vi "GUI_LeCroy64Xi.vi"() -> ()   [LabVIEW 2020]
uses:
  Shared/GUI_Template/GUI_master/tcp_new_data_event.ctl
  Shared/GUI_Template/GUI_master/tcp new data cluster.ctl
  <vilib>/Utility/miscctls.llb/LVCursorListTypeDef.ctl
  <vilib>/Utility/config.llb/Read Key (String).vi
  <vilib>/Waveform/WDTOps.llb/WDT Waveform Duration DBL.vi
  <vilib>/Analysis/NI_AAL_SigProc.lvlib
  <vilib>/measure/NI_MAPro.lvlib
  <vilib>/measure/mascope.llb/Amplitude and Levels 1 chan.vi
  <vilib>/measure/mascope.llb/Pulse Measurements 1 chan.vi
  <vilib>/Utility/config.llb/NI_LVConfig.lvlib
panel:
  in  "graph":bool
  in  "GUInumPoints::1":dbl=50000.0 caption="GUI num Points" min=100.0 max=10000.0 format="%#_6p"
  in  "TimeAxis.Time offset::1":dbl=0.0002 caption="Time offset (s)" min=-0.1 max=0.1 format="%#_6p"
  in  "Scale as scope":bool
  in  "Channel to scale":i32(ring)=1 items=["Channel 1", "Channel 2", "Channel 3", "Channel 4"]
  out "800nm w.r.t. Discharge (mean)":dbl format="%.1p"
  out "800nm w.r.t. 532nm":dbl format="%.1p"
  in  "Trigger.mode::1":u16(ring)=2 caption="Trigger mode" items=["Auto", "Normal", "Single", "Single, auto trigger"]
  in  "Trigger.Slope::1":u16(ring) caption="Trigger Slope" items=["Rising", "Falling"]
  in  "Trigger.Source::1":u16(ring)=1 caption="Trigger Source" items=["Channel 1", "Channel 2", "Channel 3", "Channel 4", "External", "Power Line"]
  in  "Trigger.Level::1":dbl=0.04 caption="Trigger Level (V)" min=0.0001 max=30.0 format="%#_6p"
  in  "TimeAxis.Max Sample Points::1":i32(ring)=5000 caption="Max Sample Points" items=["50"=50, "100"=100, "250"=250, "500"=500, "1000"=1000, "2500"=2500, "5K"=5000, "10K"=10000, "25K"=25000, "50K"=50000, "100K"=100000, "250K"=250000, "500K"=500000, "1M"=1000000, "2M"=2000000, "2.5M"=2500000, "5M"=5000000, "10M"=10000000, "25M"=25000000, "50M"=50000000, "100M"=100000000]
  in  "TimeAxis.Time base::1":dbl=0.0002 caption="Time base (s/div)" min=2e-10 max=1000.0 format="%#_6p"
  in  "Chenabled.Channel2::1":bool=TRUE caption="On/Off"
  in  "Verticaloffset.Channel2::1":dbl caption="Vertical Offset (V)" min=-40.0 max=40.0 format="%#.6p"
  in  "Bandwidth.Channel2::1":u16(ring) caption="Bandwidth" items=["Full", "20MHZ", "200MHZ"]
  in  "Verticalrange.Channel2::1":dbl=0.2 caption="Vertical Range (V)" min=0.0001 max=80.0 format="%#.6p"
  in  "Chenabled.Channel3::1":bool caption="On/Off"
  in  "Verticaloffset.Channel3::1":dbl caption="Vertical Offset (V)" min=-40.0 max=40.0 format="%#.6p"
  in  "Bandwidth.Channel3::1":u16(ring) caption="Bandwidth" items=["Full", "20MHZ", "200MHZ"]
  in  "Verticalrange.Channel3::1":dbl=0.2 caption="Vertical Range (V)" min=0.0001 max=80.0 format="%#.6p"
  in  "timeout::1":dbl caption="Timeout (ms)" min=0.0 max=10.0
  in  "Tab Control":T1(tab)
  out "all traces":waveform(dbl)[](graph)
  in  "value6::2":dbl=1.07e-07 caption="Dischage output" min=-9999999.0 max=9999999.0 step=1e-09 format="%#_6p"
  in  "value5::2":dbl=6e-08 caption="Dischage input" min=-9999999.0 max=9999999.0 step=1e-09 format="%#_6p"
  in  "value4::2":dbl=3e-09 caption="800nm diode" min=-9999999.0 max=9999999.0 step=1e-09 format="%#_6p"
  in  "value3::2":dbl caption="532nm diode" min=-9999999.0 max=9999999.0 step=1e-09 format="%#_6p"
  in  "Digitizer Traces":T2 caption="Raw Scope Data"
  in  "Type":enum16{"Peak fit", "Threshold"}[](array[ring])=[enum."Peak fit", enum."Threshold", enum."Peak fit", enum."Peak fit"]
  in  "Fit width":i32[](array[numeric])=[13, 15, 2000, 2000] min=3
  in  "Fit threshold":dbl[](array[numeric])=[0.02, 0.01, 0.02, 0.02]
  in  "Enable fitting":bool=TRUE
  in  "Enable fit cursors":bool=TRUE
  out "Number of peaks found":i32[](array[numeric])
  out "Time of peak":dbl[](array[numeric]) format="%.2p"
  in  "CH 4:":bool=TRUE
  in  "CH 3:":bool=TRUE
  in  "CH 2:":bool
  in  "CH 1:":bool
  in  "GUIdevice 1":string="LeCroy8254M"
  in  "GUIdevice 2":string="Offsets-Timing"
  out "error IO 2":errorcluster
  out "error":errorcluster
  out "tcp data event":T3
  out "duration":dbl format="%.2p"
  in  "Fit parameters file path":string="user data\\LeCroy_Fit_Parameters.txt"
  in  "stop":bool
  in  "Chenabled.Channel1::1":bool=TRUE caption="On/Off"
  in  "Verticaloffset.Channel1::1":dbl caption="Vertical Offset (V)" min=-5.0 max=5.0 format="%#.6p"
  in  "Bandwidth.Channel1::1":u16(ring) caption="Bandwidth" items=["Full", "20MHZ", "200MHZ"]
  in  "Verticalrange.Channel1::1":dbl=1.2 caption="Vertical Range (V)" min=0.0001 max=80.0 format="%#.6p"
  in  "Chenabled.Channel0::1":bool caption="On/Off"
  in  "Verticaloffset.Channel0::1":dbl caption="Vertical Offset (V)" min=-5.0 max=5.0 format="%#.6p"
  in  "Bandwidth.Channel0::1":u16(ring) caption="Bandwidth" items=["Full", "20MHZ", "200MHZ"]
  in  "Verticalrange.Channel0::1":dbl=0.2 caption="Vertical Range (V)" min=0.0001 max=80.0 format="%#.6p"
  # "Scope controls"
  # "Time axis"
  # "Scaling"
  # "Raw"
  # "Converted"
  # "Trigger"
  # "Channel 3"
  # "Channel 4"
  # "time offsets"
  # "time offsets"
  # "Fit settings"
  # "CH 1"
  # "CH 2"
  # "CH 3"
  # "CH 4"
  # "Fit output"
  # "CH 1"
  # "CH 2"
  # "CH 3"
  # "CH 4"
  # "Channel 2"
  # "Channel 1"
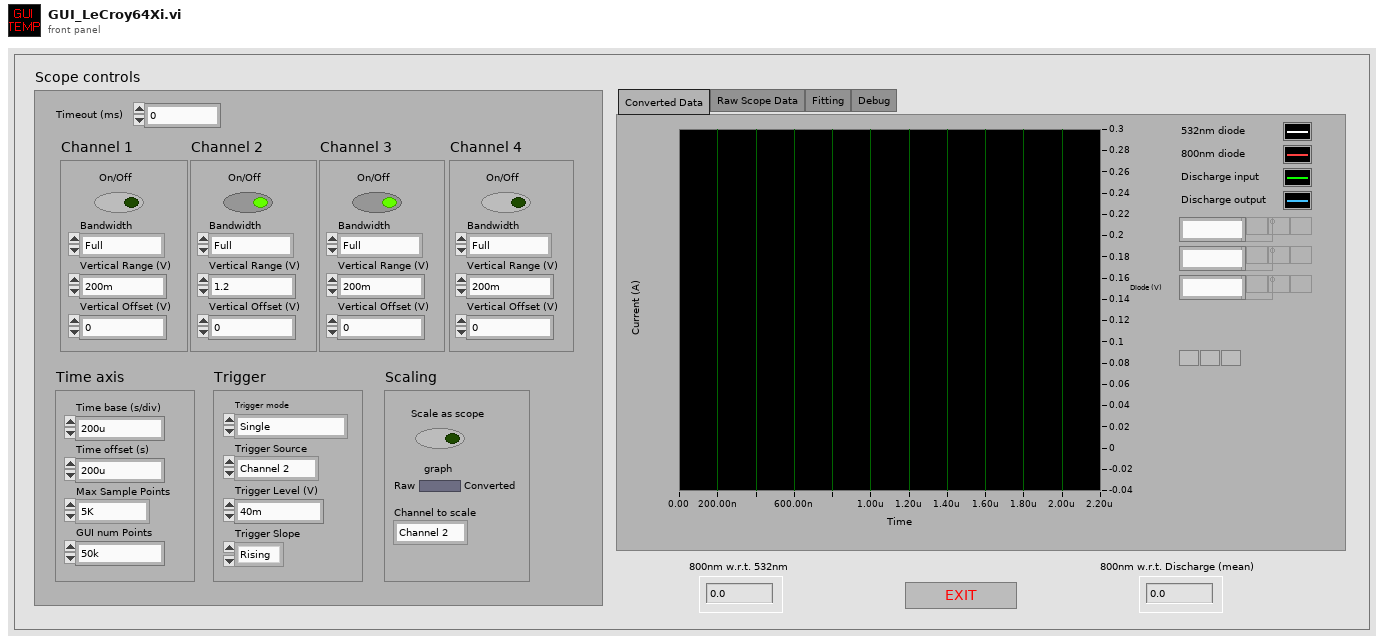
[diagram p1: front panel]
types:
  T1 = enum32{"Converted Data", "Raw Scope Data", "Fitting", "Debug"}
  T2 = cluster{"Channel::1":enum16{"Channel0", "Channel1", "Channel2", "Channel3"}, "scopeTraceGUI::1":waveform(dbl)[]}
  T3 = typedef "tcp_new_data_event.ctl" = refnum<user-event>
  T4 = typedef "tcp new data cluster.ctl" = cluster{"EventEnum":enum16{"new data", "connection status update"}, "Device name":string}
  T5 = enum32{"invalid app kind", "Development System", "Run Time System", "Student Edition", "Embedded LabVIEW", "Evaluation", "Custom"}
  T6 = enum32{"Invalid", "Standard", "Closed", "Hidden", "Minimized", "Maximized"}
  T7 = typedef "LVCursorListTypeDef.ctl" = cluster{"Name":string, "Color":u32, "Style":u8, "Point Style":u8, "Name Visible":bool, "Allow Drag":bool, "Cursor Mode":u32, "Plot":i32, "Index":i32, "Position":cluster{"X":dbl, "Y":dbl}, "X Scale":u32, "Y Scale":u32, "Watch Plots":i32[], "Watch All Plots":bool, "Plot Area":i32, "Label Offset":cluster{"X":dbl, "Y":dbl}}[]
  T8 = cluster{"Core":cluster{"Current VI Reference":refnum<vi>, "Close Panel on Exit?":bool}, "scopeTraceGUI::1":waveform(dbl)[], "Display Error Popup":bool, "time offsets":dbl[], "initilize fit":bool, "Fit peaks":dbl[], "fit cursors enabled":bool, "fitting enabled":bool}
  T9 = cluster{"Current VI Reference":refnum<vi>, "Close Panel on Exit?":bool}
  T10 = typedef "NI_LVConfig.lvlib/Config Data RefNum.ctl" = refnum<k1>
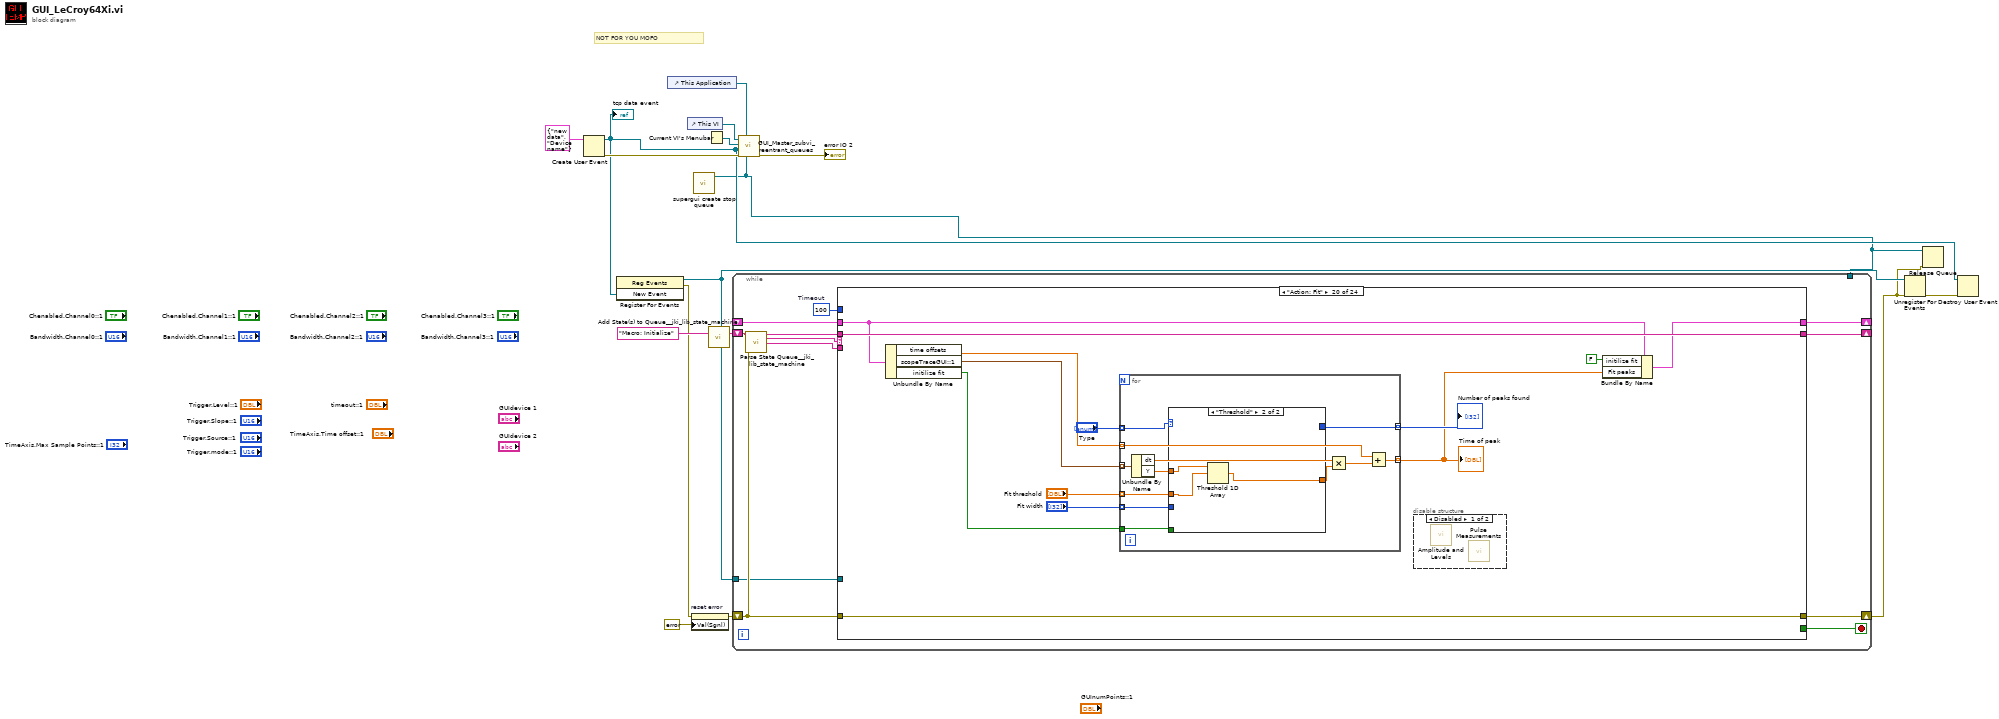
[diagram p0: block diagram]
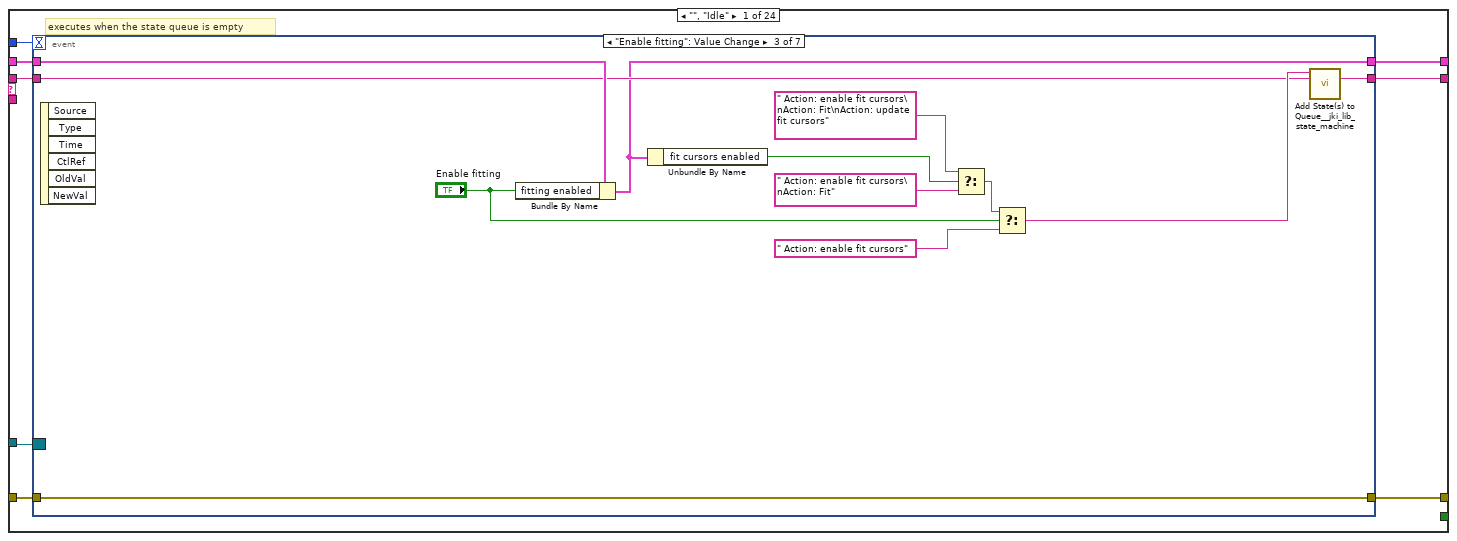
[diagram p2: hidden frame]
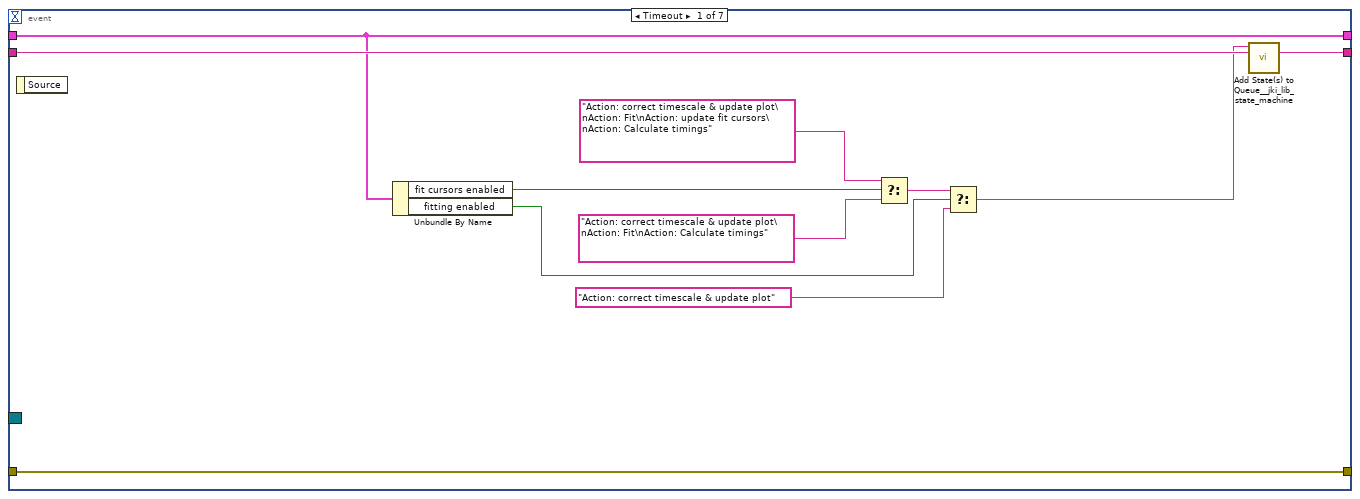
[diagram p3: hidden frame]
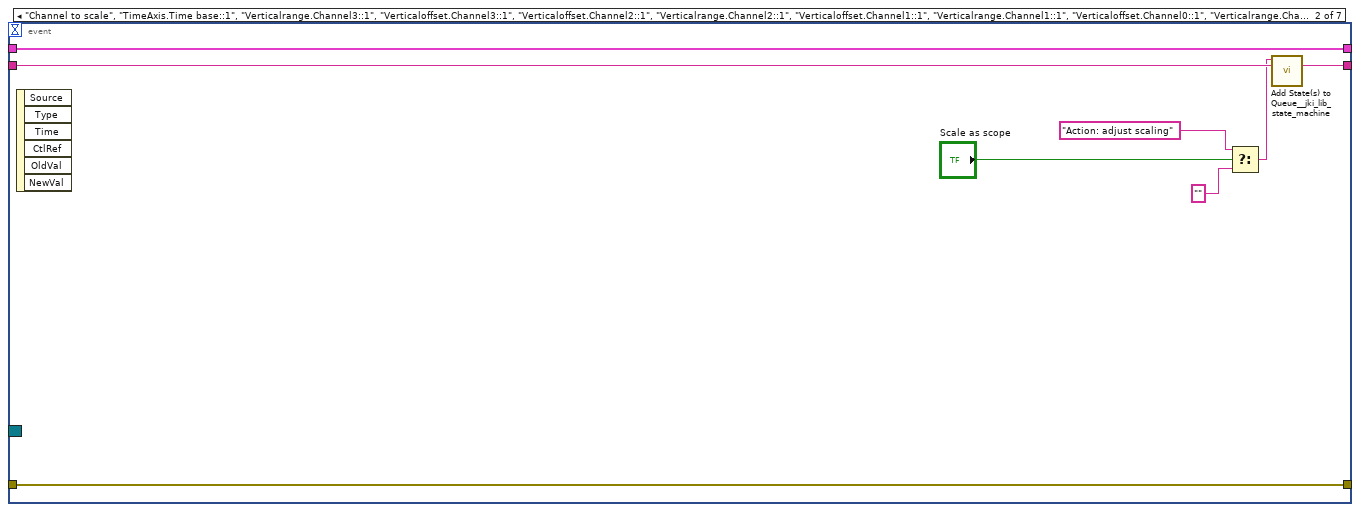
[diagram p4: hidden frame]
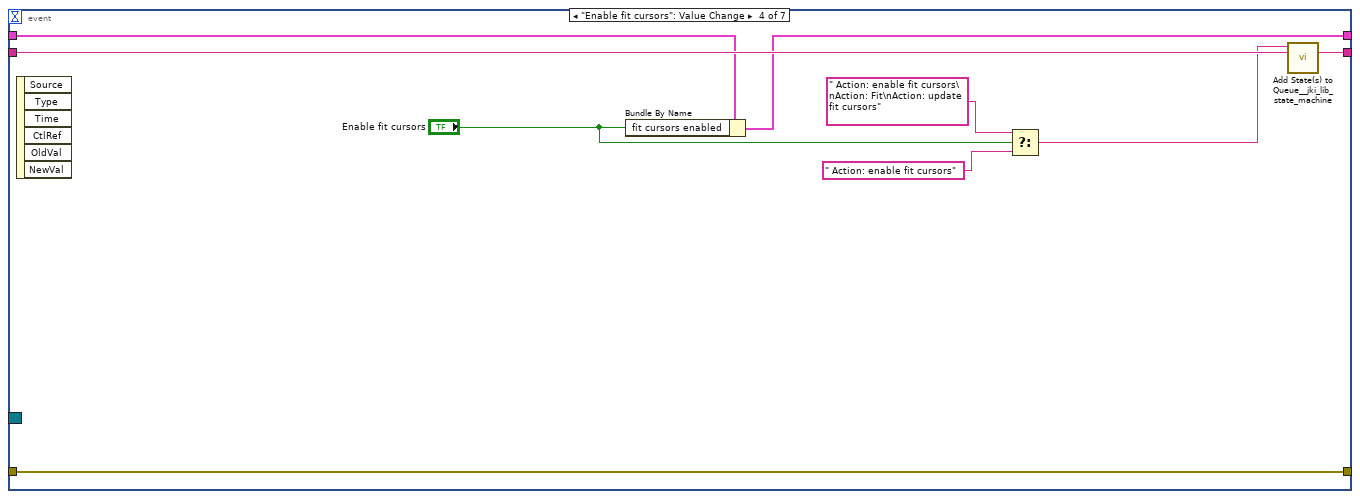
[diagram p5: hidden frame]
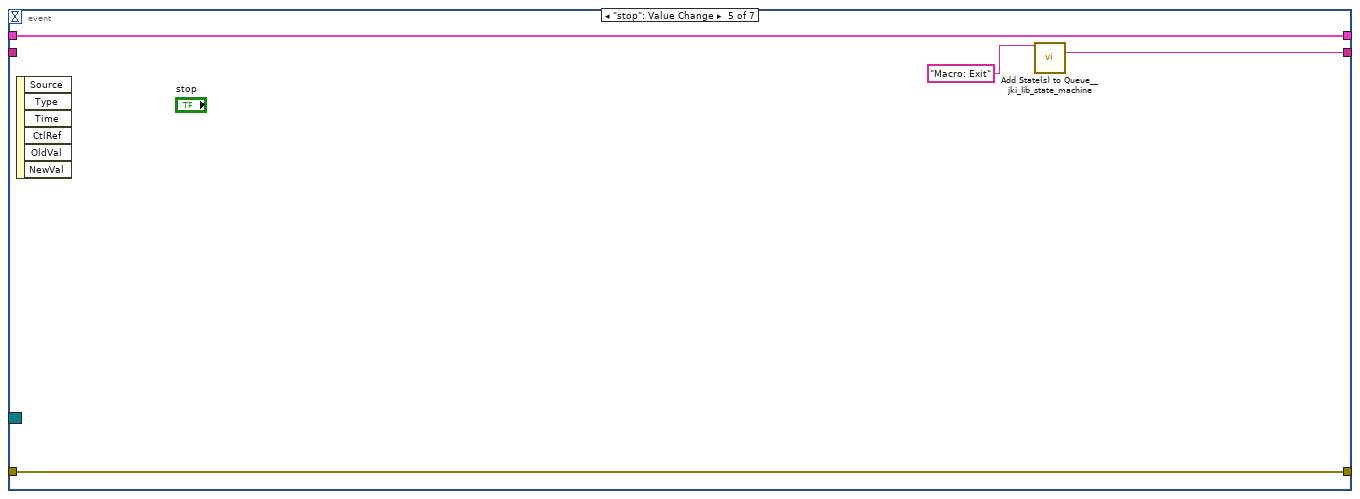
[diagram p6: hidden frame]
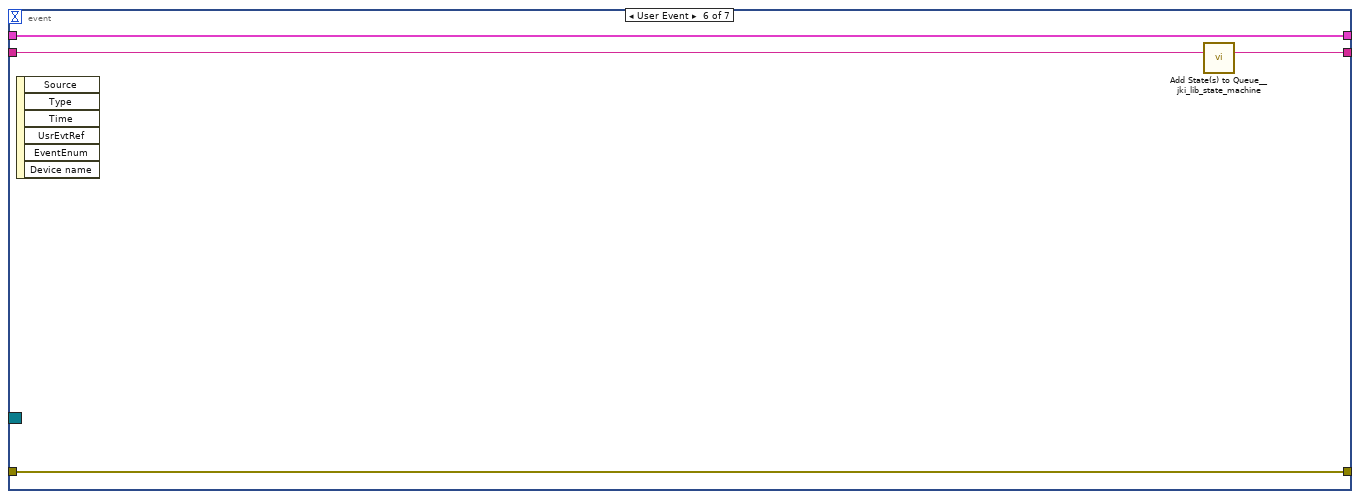
[diagram p7: hidden frame]
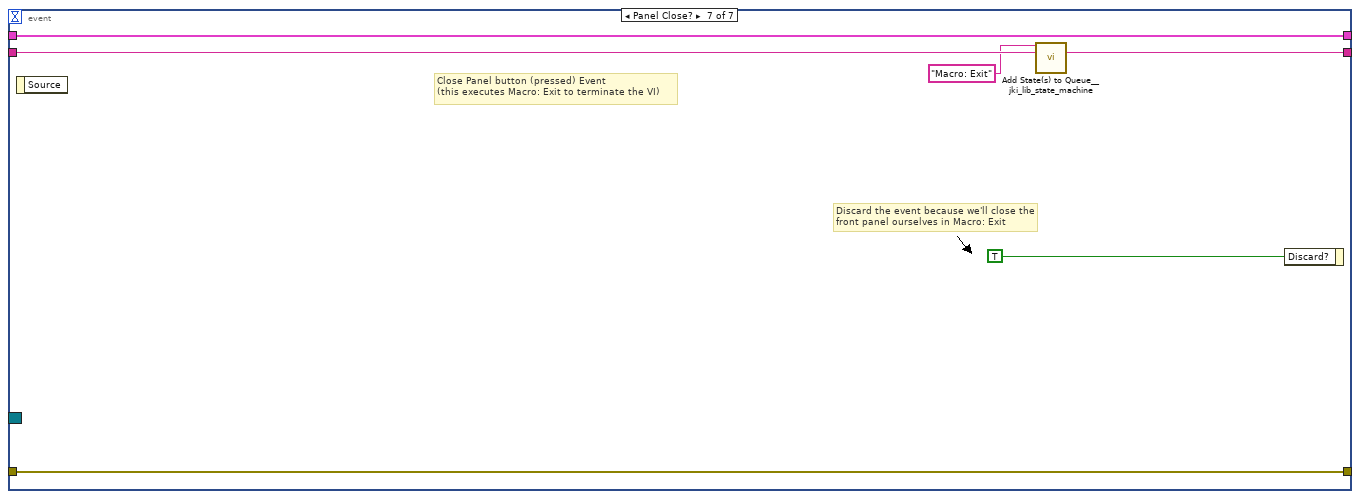
[diagram p8: hidden frame]
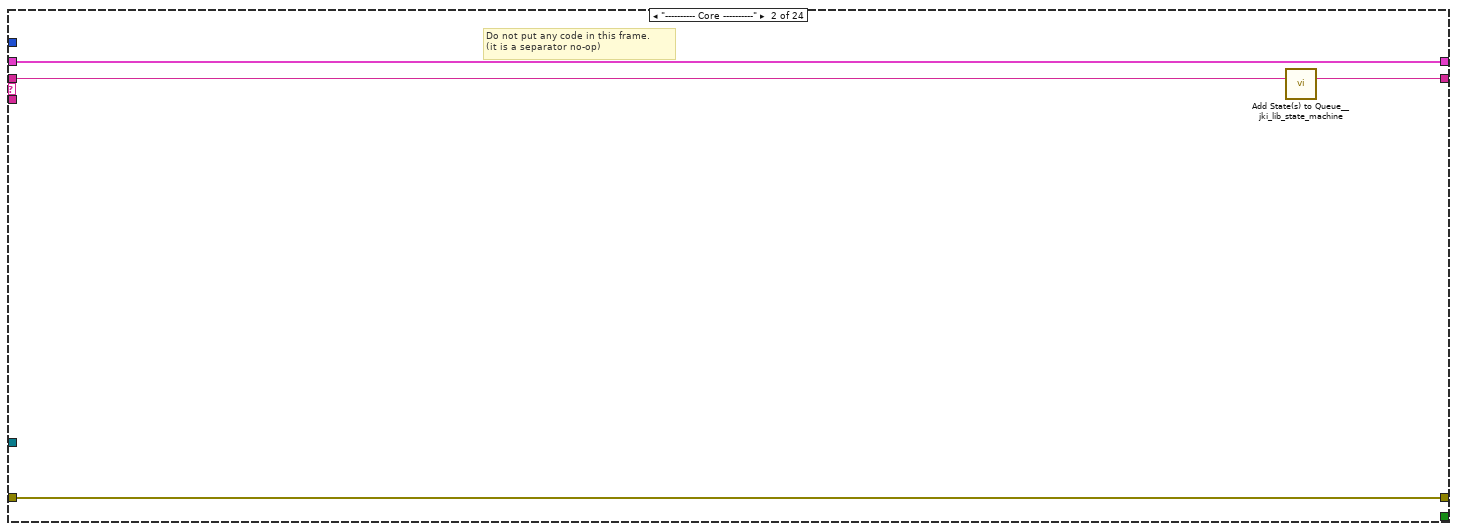
[diagram p9: hidden frame]
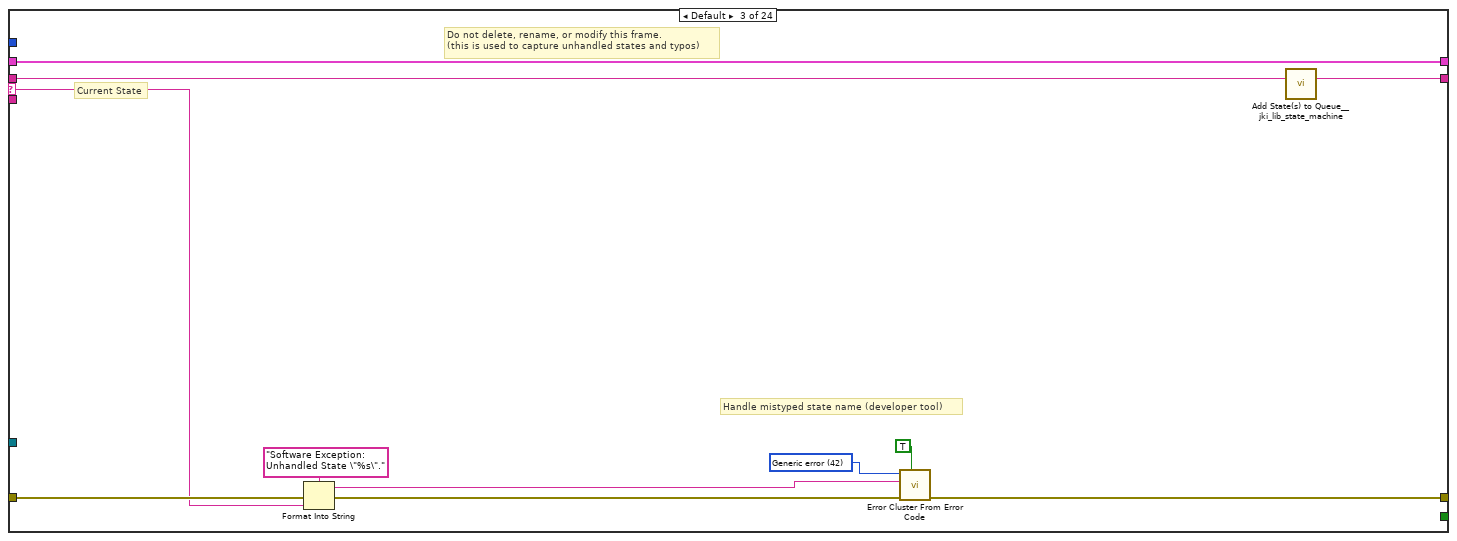
[diagram p10: hidden frame]
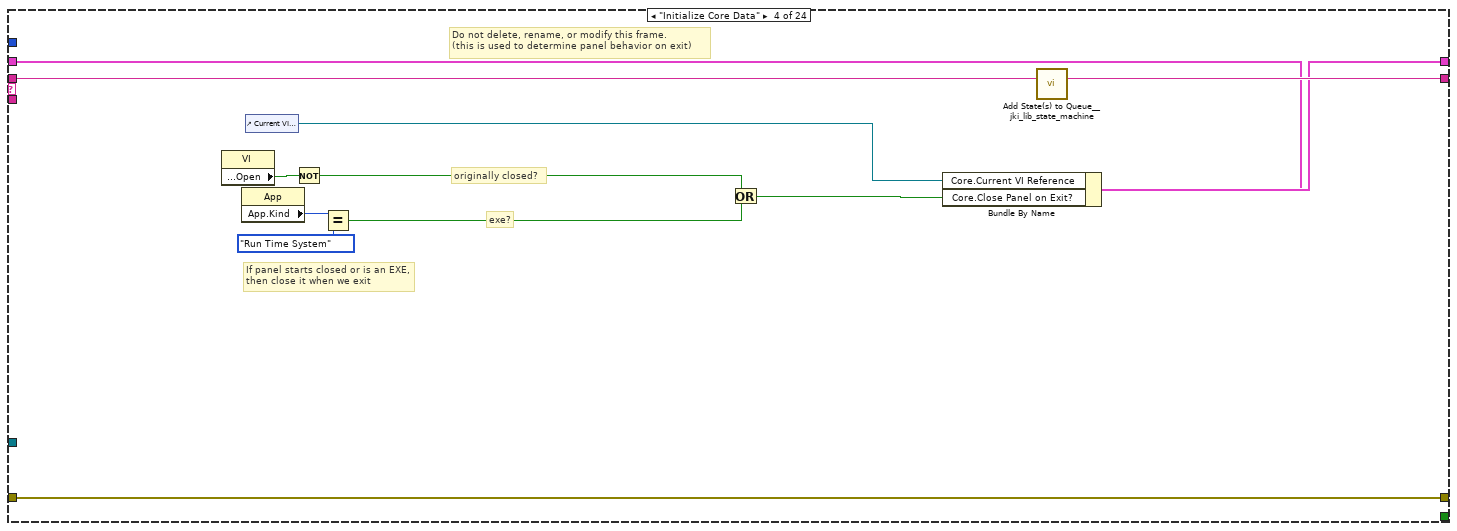
[diagram p11: hidden frame]
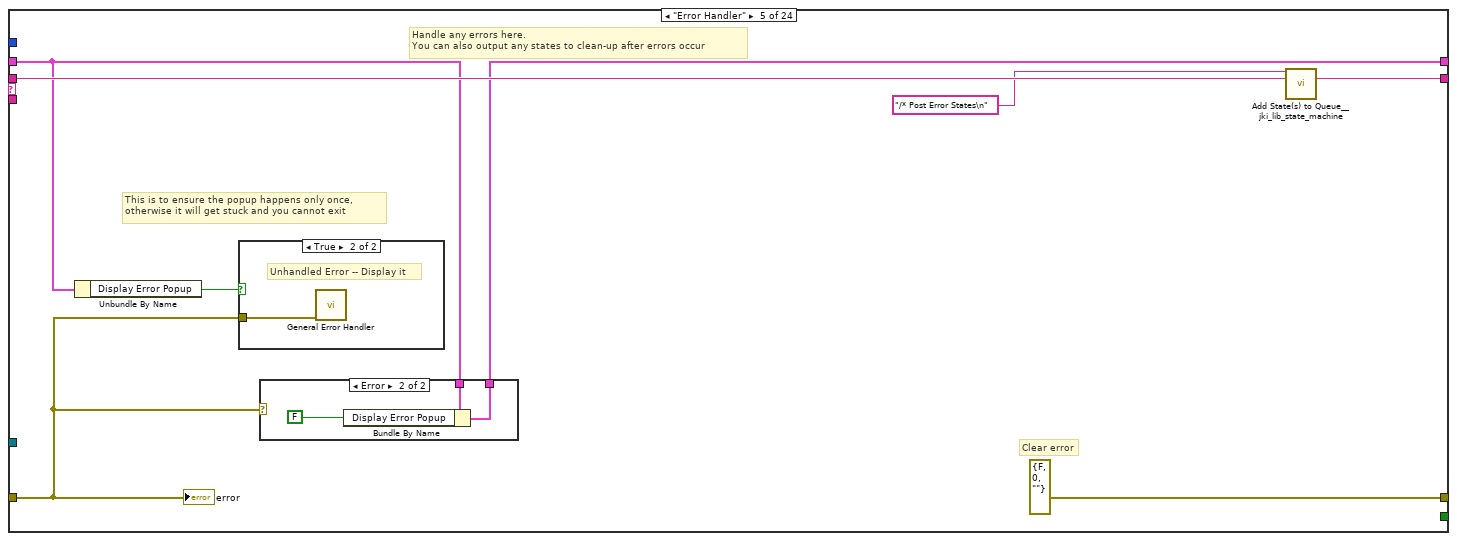
[diagram p12: hidden frame]
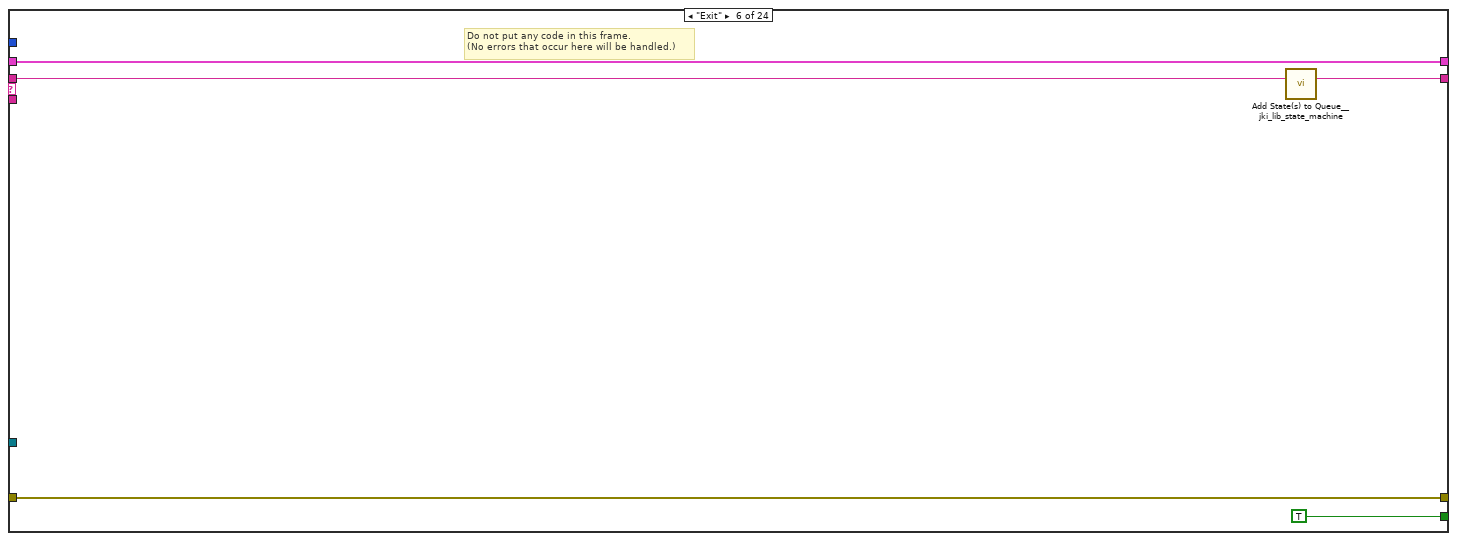
[diagram p15: hidden frame]
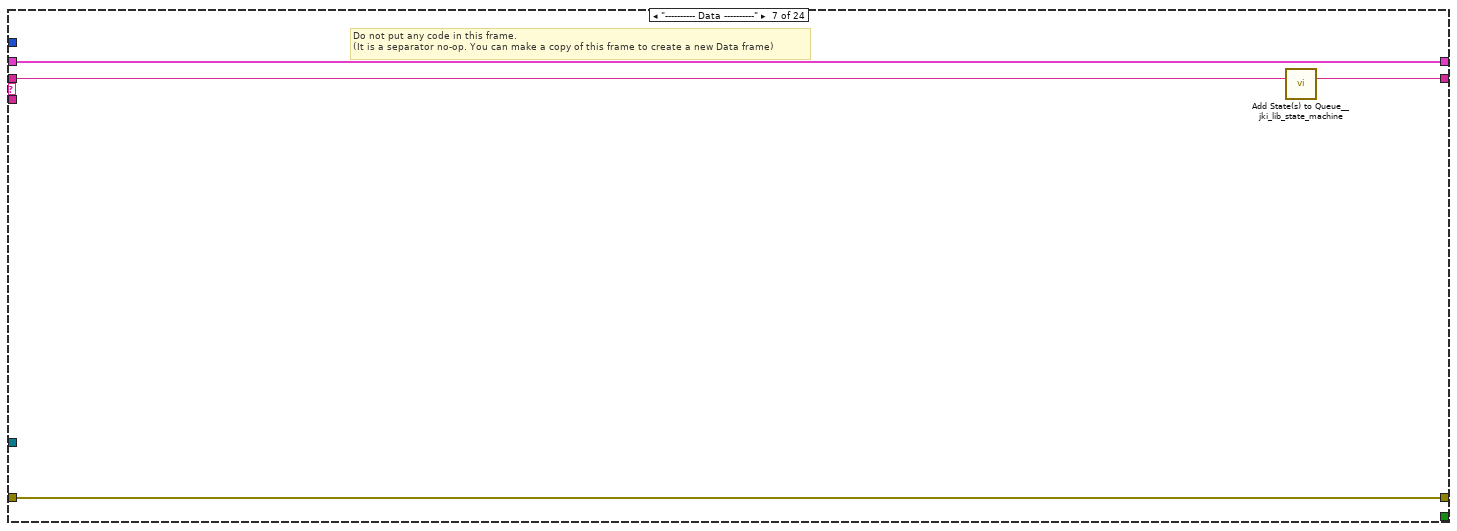
[diagram p16: hidden frame]
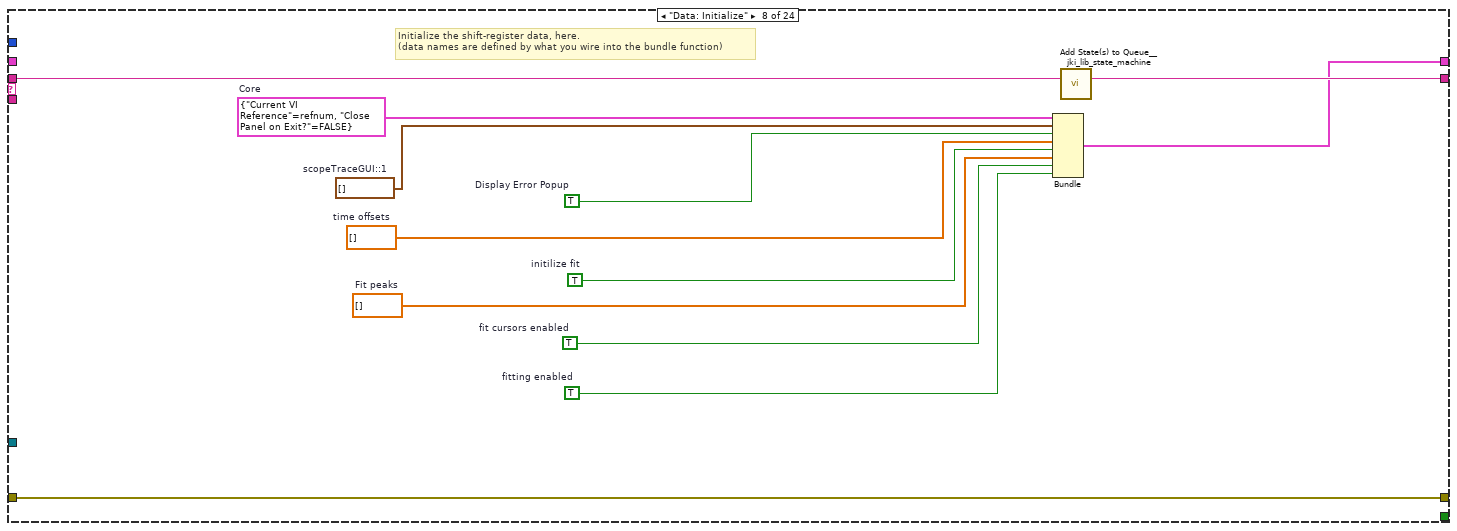
[diagram p17: hidden frame]
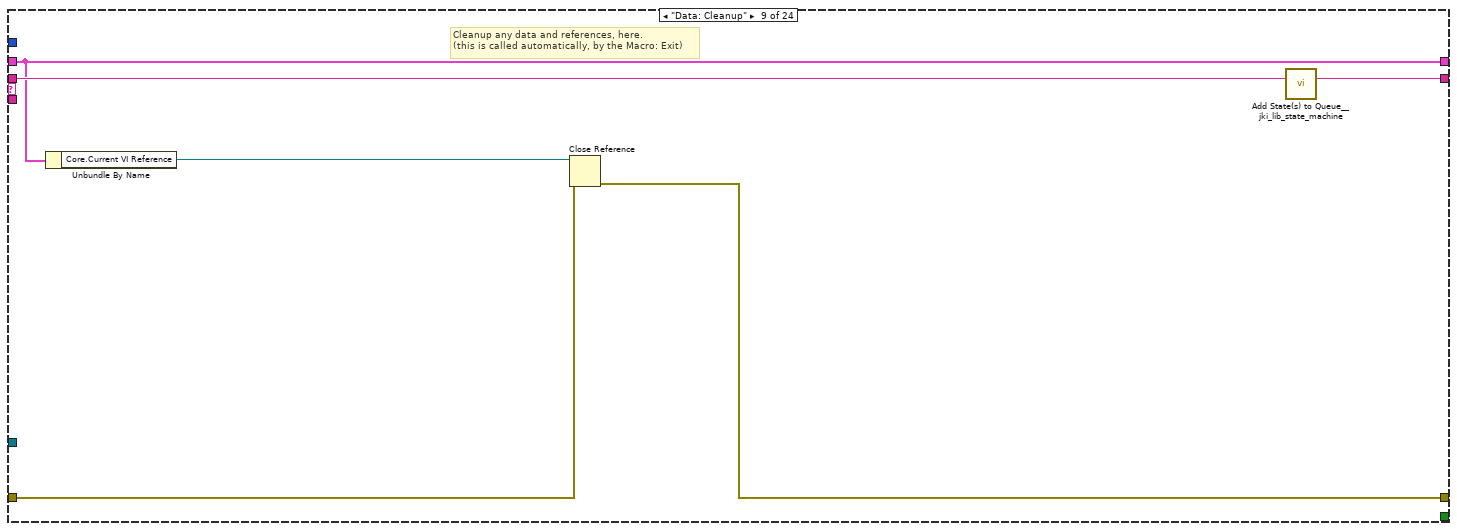
[diagram p18: hidden frame]
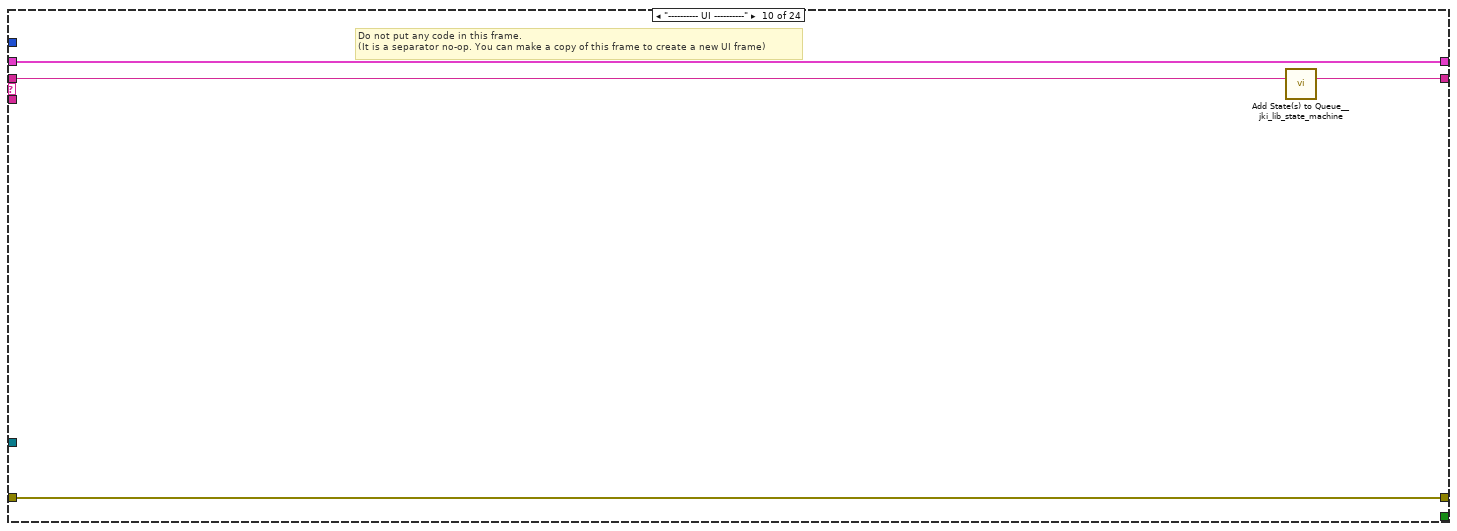
[diagram p19: hidden frame]
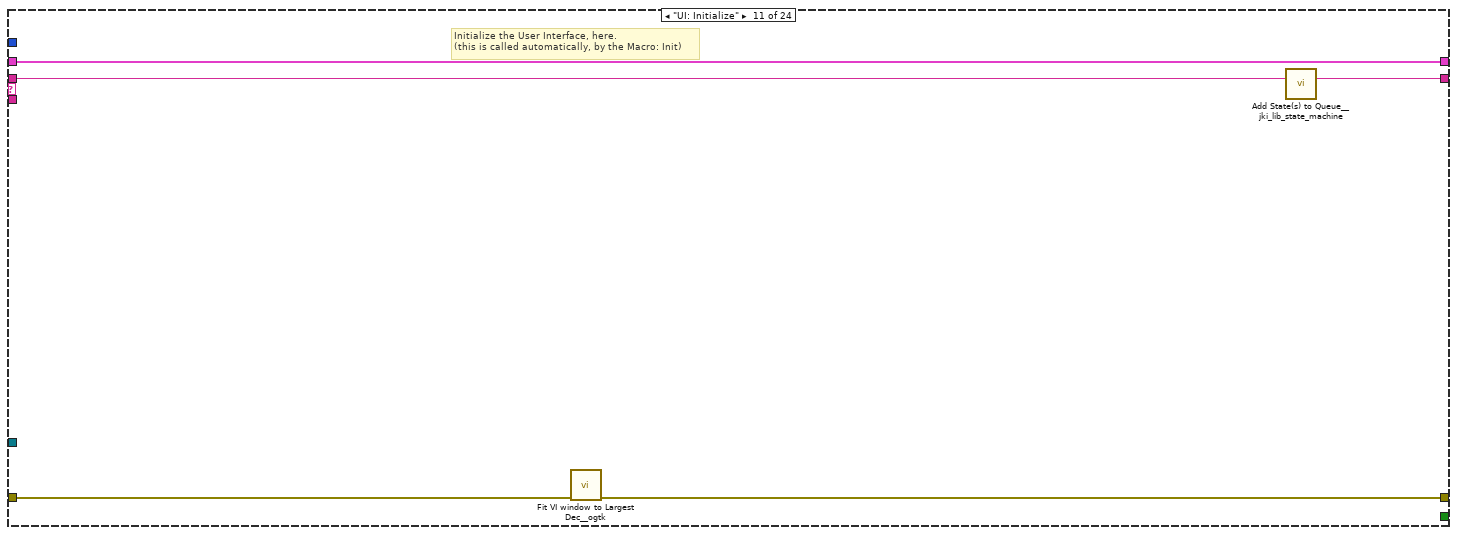
[diagram p20: hidden frame]
diagram:
  # "NOT FOR YOU MOFO"
  n1 = Create User Event(user event datatype=T4 {"EventEnum"=enum."new data", "Device name"="Device name"} ("New Event")) -> (user event=w10:refnum<user-event>, error out=w12:errorcluster)  [unwired: 1 in]
  "tcp data event" <- w10
  n2 = register-events(w10) -> (reference out=w7:refnum<event-registration>, error out=w1:errorcluster)  [unwired: 2 in]
  n3 = control-ref of="This Application"() -> (w11:refnum<vi>)
  n4 = control-ref of="This VI"() -> (w15:refnum<vi>)
  n5 = property on="reset error" class="Clust (strict)"(error in=w1, "Val(Sgnl)"=errorcluster {"status"=FALSE, "code"=0, "source"=""} ("Value (Signaling)")) -> (error out=w2:errorcluster)  [unwired: 1 in, 1 out]
  n6 = call "supergui create stop queue.vi"() -> ("STOP Queue out"=w6:refnum<queue>)  [unwired: 11 in]
  n7 = Current VI's Menubar() -> (w14:refnum<k9>)
  n8 = call <vilib>:"Add State(s) to Queue__jki_lib_state_machine.vi"("State(s) in (\"\")"="Macro: Initialize") -> ("States Out"=w9:string)  [unwired: 14 in]
  n9 = while "JKI - String-Based Queued State Machine (Basic) v1.0" {
    shift-right: [w21] -> _
    shift-left: _ -> [w20]
    shift-right: [w24] -> w4
    shift-left: w2 -> [w18]
    shift-right: [w23] -> _
    shift-left: w9 -> [w25]
    tunnel: w7 -> [w17]
    tunnel: w6 -> [_]
    stop <- w22 stop-if-true
    w19 = 100  # Timeout
    n10 = call <vilib>:"Parse State Queue__jki_lib_state_machine.vi"("State Queue"=w25, "Error In (no error)"=w18) -> ("Remaining States"=w27:string, "Current State"=w28:string, "Arguments"=w26:string)  [unwired: 11 in]
    n11 = case shown="\"Action: Fit\"" w28 {
      selector: w28 -> [_ _ w95 _ _ _ _ _ _ _ _ _ _ _ _ _ _ _ _ _ _ _ _ _]
      tunnel: w27 -> [w36 w94 w99 w117 w125 w135 w139 w151 w157 w161 w166 w235 w243 w254 w280 w285 w295 w299 w314 w346 w377 w388 w407 w426]
      tunnel: w26 -> [_ _ _ _ _ _ _ _ _ _ _ _ w238 w248 _ _ _ _ _ _ _ _ _ _]
      tunnel: w20 -> [w34 w91 w97 w108 w119 w133 w136 _ w152 w158 w164 w233 w241 w250 w277 w282 w293 w296 w302 w341 w375 w387 w406 w427]
      tunnel: [w33 w92 w101 w114 errorcluster {"status"=FALSE, "code"=0, "source"=""} ("error out") w132 w137 w148 w153 w159 w162 w216 w239 w251 w278 w283 w286 w297 w310 w347 w373 w389 w408 w428] -> w24
      tunnel: w18 -> [w32 w92 w100 w114 w121 w132 w137 w148 w154 w159 w163 w215 w240 w252 w278 w283 w286 w297 w311 w347 w374 w384 w408 w411]
      tunnel: [w35 w93 w98 w116 w124 w134 w138 w150 w156 w160 w165 w234 w242 w253 w279 w284 w294 w298 w313 w346 w377 w388 w407 w426] -> w23
      tunnel: [_ _ _ _ _ TRUE _ _ _ _ _ _ _ _ _ _ _ _ _ _ _ _ _ _] -> w22
      tunnel: [w31 w91 w97 w115 w118 w133 w136 w149 w152 w158 w164 w233 w241 w250 w277 w282 w293 w296 w312 w340 w375 w387 w406 w427] -> w21
      tunnel: w19 -> [w30 _ _ _ _ _ _ _ _ _ _ _ _ _ _ _ _ _ _ _ _ _ _ _]
      tunnel: w17 -> [w29 _ _ _ _ _ _ _ _ _ _ _ _ _ _ _ _ _ _ _ _ _ _ _]
      frame "", "Idle" {
        # "executes when the state queue is empty"
        n12 = event shown="[2] \"Enable fitting\": Value Change" {
          selector: w29 -> [_ _ _ _ _ _ _]
          dyn-events: _ -> [_ _ _ _ _ _ _]
          timeout: w30 -> [_ _ _ _ _ _ _]
          tunnel: w36 -> [w47 w54 w62 w74 _ w82 w90]
          tunnel: [w46 w55 w63 w75 w78 w83 w89] -> w35
          tunnel: w34 -> [w42 w53 w66 w73 w80 w81 w87]
          tunnel: [w45 w52 w67 w76 w77 w84 w88] -> w33
          tunnel: w32 -> [w45 w52 w67 w76 w77 w84 w88]
          tunnel: [w42 w53 w60 w72 w80 w81 w87] -> w31
          event Timeout {
            n13 = event-data() -> ()  [unwired: 1 in, 1 out]
            n14 = Unbundle By Name(w42) -> ("fit cursors enabled"=w41:bool, "fitting enabled"=w37:bool)
            n15 = Select(t="Action: correct timescale & update plot\nAction: Fit\nAction: update fit cursors\nAction: Calculate timings" ("State(s) in Front (\"\")"), s=w41, f="Action: correct timescale & update plot\nAction: Fit\nAction: Calculate timings" ("State(s) in Front (\"\")")) -> (s? t:f=w40:string)
            n16 = Select(t=w40, s=w37, f="Action: correct timescale & update plot" ("State(s) in Front (\"\")")) -> (s? t:f=w39:string)
            n17 = call <vilib>:"Add State(s) to Queue__jki_lib_state_machine.vi"("State(s) in Front (\"\")"=w39, "State(s) in (\"\")"=w47) -> ("States Out"=w46:string)  [unwired: 13 in]
          }
          event "Channel to scale", "TimeAxis.Time base::1", "Verticalrange.Channel3::1", "Verticaloffset.Channel3::1", "Verticaloffset.Channel2::1", "Verticalrange.Channel2::1", "Verticaloffset.Channel1::1", "Verticalrange.Channel1::1", "Verticaloffset.Channel0::1", "Verticalrange.Channel0::1", "Scale as scope", "graph": Value Change {
            n18 = event-data() -> ()  [unwired: 1 in, 6 out]
            n19 = Select(t="Action: adjust scaling", s="Scale as scope", f="") -> (s? t:f=w51:string)
            n20 = call <vilib>:"Add State(s) to Queue__jki_lib_state_machine.vi"("State(s) in Front (\"\")"=w51, "State(s) in (\"\")"=w54) -> ("States Out"=w55:string)  [unwired: 13 in]
          }
          event "Enable fitting": Value Change {
            n21 = event-data() -> ()  [unwired: 1 in, 6 out]
            n22 = Bundle By Name(cluster=w66, "fitting enabled"="Enable fitting") -> (w60:T8)
            n23 = Unbundle By Name(w60) -> ("fit cursors enabled"=w56:bool)
            n24 = Select(t=" Action: enable fit cursors\nAction: Fit\nAction: update fit cursors" ("State(s) in Front (\"\")"), s=w56, f=" Action: enable fit cursors\nAction: Fit" ("State(s) in Front (\"\")")) -> (s? t:f=w59:string)
            n25 = Select(t=w59, s="Enable fitting", f=" Action: enable fit cursors" ("State(s) in Front (\"\")")) -> (s? t:f=w65:string)
            n26 = call <vilib>:"Add State(s) to Queue__jki_lib_state_machine.vi"("State(s) in Front (\"\")"=w65, "State(s) in (\"\")"=w62) -> ("States Out"=w63:string)  [unwired: 13 in]
          }
          event "Enable fit cursors": Value Change {
            n27 = event-data() -> ()  [unwired: 1 in, 6 out]
            n28 = Bundle By Name(cluster=w73, "fit cursors enabled"="Enable fit cursors") -> (w72:T8)
            n29 = Select(t=" Action: enable fit cursors\nAction: Fit\nAction: update fit cursors" ("State(s) in Front (\"\")"), s="Enable fit cursors", f=" Action: enable fit cursors" ("State(s) in Front (\"\")")) -> (s? t:f=w71:string)
            n30 = call <vilib>:"Add State(s) to Queue__jki_lib_state_machine.vi"("State(s) in Front (\"\")"=w71, "State(s) in (\"\")"=w74) -> ("States Out"=w75:string)  [unwired: 13 in]
          }
          event "stop": Value Change {
            n31 = event-data() -> ()  [unwired: 1 in, 6 out]
            n32 = call <vilib>:"Add State(s) to Queue__jki_lib_state_machine.vi"("State(s) in Front (\"\")"="Macro: Exit") -> ("States Out"=w78:string)  [unwired: 14 in]
          }
          event User Event {
            n33 = event-data() -> ()  [unwired: 1 in, 6 out]
            n34 = call <vilib>:"Add State(s) to Queue__jki_lib_state_machine.vi"("State(s) in (\"\")"=w82) -> ("States Out"=w83:string)  [unwired: 14 in]
          }
          event Panel Close? {
            # "Discard the event because we'll close the front panel ourselves in Macro: Exit"
            # "Close Panel button (pressed) Event\n(this executes Macro: Exit to terminate the VI)"
            n35 = event-data() -> ()  [unwired: 1 in, 1 out]
            n36 = call <vilib>:"Add State(s) to Queue__jki_lib_state_machine.vi"("State(s) in Front (\"\")"="Macro: Exit", "State(s) in (\"\")"=w90) -> ("States Out"=w89:string)  [unwired: 13 in]
            n37 = event-data("Discard?"=TRUE) -> ()  [unwired: 1 in, 1 out]
          }
        }
      }
      frame "---------- Core ----------" {
        # "Do not put any code in this frame.\n(it is a separator no-op)"
        n38 = call <vilib>:"Add State(s) to Queue__jki_lib_state_machine.vi"("State(s) in (\"\")"=w94) -> ("States Out"=w93:string)  [unwired: 14 in]
      }
      frame Default {
        w104 = 42 items=["No error", "Argument error", "Memory is full", "Out of zone", "End of file", "File already open", "Generic file I/O error", "File not found", "File permission error", "Disk is full", "Duplicate path", "Too many files open", "System feature not enabled", "Resource file not found", "Cannot add resource", "Resource not found", "Image not found", "Image memory error", "Pen does not exist", "Config type invalid", "Config token not found", "Config parse error", "Config memory error", "Bad external code format", "Bad external code offset", "External code not present", "Null window", "Destroy window error", "Null menu", "Print aborted", "Bad print record", "Print driver error", "Windows error during printing", "Memory error during printing", "Print dialog error", "Generic print error", "Invalid device refnum", "Device not found", "Device parameter error", "Device unit error", "Cannot open device", "Device call aborted", "Generic error", "Cancelled by user", "Object ID too low", "Object ID too high", "Object not in heap", "Unknown heap", "Unknown object (invalid DefProc)", "Unknown object (DefProc not in table)", "Message out of range", "Invalid (null) method", "Unknown message", "Manager call not supported", "Bad address", "Network operation in progress", "Network operation timed out", "Connection is busy", "Network attribute not supported", "Network error", "Address in use", "System out of memory", "Connection aborted", "Connection refused", "Not connected", "Already connected", "Connection closed", "Initialization error (interapplication manager)", "Bad occurrence", "Wait on unbound occurrence handler", "Occurrence queue overflow", "Datalog type conflict", "Unused", "Unrecognized type (interapplication manager)", "Memory corrupt", "Failed to make temporary DLL", "Old CIN version", "Drag socket not found", "Failed to load drop-object", "Failed to register OLE object", "Failed to release OLE object", "Format specifier type mismatch", "Unknown format specifier", "Too few format specifiers", "Too many format specifiers", "Scan failed", "Newer CIN version", "Error converting to variant", "Runtime menu error", "Password tampered", "Variant attribute not found", "Incompatible variant data type", "Event data is not available", "Event Store is not present", "Occurrence is not found", "Event Queue is not created", "Event info is not available", "Refnum passed is NULL", "Error retrieving Class GUID", "Error retrieving CoClass GUID", "Error retrieving TypeLib GUID.", "Bad built application magic bytes.", "Specific driver is different from the specific driver associated with the Logical Name.", "There is no session opened to the class driver.", "Max Error", "MAX - Error with config objects", "MAX - Error loading configuration", "MAX - Group not supported"]
        # "Current State"
        # "Do not delete, rename, or modify this frame.\n(this is used to capture unhandled states and typos)"
        # "Handle mistyped state name (developer tool)"
        n39 = Format Into String(format string="Software Exception: Unhandled State \"%s\"." ("message"), error in=w100, w95) -> (resulting string=w103:string, error out=w102:errorcluster)  [unwired: 1 in]
        n40 = call <vilib>:"Error Cluster From Error Code.vi"("show call chain? (False)"=TRUE, "error in (no error)"=w102, "error message (\"\")"=w103, "error code (0)"=w104) -> ("error out"=w101:errorcluster)  [unwired: 5 in]
        n41 = call <vilib>:"Add State(s) to Queue__jki_lib_state_machine.vi"("State(s) in (\"\")"=w99) -> ("States Out"=w98:string)  [unwired: 14 in]
      }
      frame "Initialize Core Data" {
        # "Do not delete, rename, or modify this frame.\n(this is used to determine panel behavior on exit)"
        # "originally closed?"
        # "exe?"
        # "If panel starts closed or is an EXE, then close it when we exit"
        n42 = property class="VI"() -> ("Front Panel.Open"=w113:bool)  [unwired: 2 in, 2 out]
        n43 = property class="App"() -> ("App.Kind"=w112:T5)  [unwired: 2 in, 2 out]
        n44 = control-ref of="Current VI Reference"() -> (w106:refnum<vi>)
        n45 = Not(x=w113) -> (.not. x?=w110:bool)
        n46 = Equal?(x=w112, y=T5."Run Time System" ("Application:Kind")) -> (x = y?=w109:bool)
        n47 = Or(x=w110, y=w109) -> (x .or. y?=w107:bool)
        n48 = Bundle By Name(cluster=w108, "Core.Current VI Reference"=w106, "Core.Close Panel on Exit?"=w107) -> (w115:T8)
        n49 = call <vilib>:"Add State(s) to Queue__jki_lib_state_machine.vi"("State(s) in (\"\")"=w117) -> ("States Out"=w116:string)  [unwired: 14 in]
      }
      frame "Error Handler" {
        # "This is to ensure the popup happens only once, \notherwise it will get stuck and you cannot exit"
        # "Handle any errors here.\nYou can also output any states to clean-up after errors occur"
        # "Clear error"
        n50 = Unbundle By Name(w119) -> ("Display Error Popup"=w120:bool)
        n51 = case shown="True" w120 {
          tunnel: w121 -> [_ w126]
          frame False {
          }
          frame True {
            # "Unhandled Error -- Display it"
            n52 = call <vilib>:"General Error Handler.vi"("error in (no error)"=w126) -> ()  [unwired: 10 in, 5 out]
          }
        }
        n53 = case shown="Error" w121 {
          tunnel: w119 -> [w127 w130]
          tunnel: [w127 w129] -> w118
          frame No Error {
          }
          frame Error {
            n54 = Bundle By Name(cluster=w130, "Display Error Popup"=FALSE) -> (w129:T8)
          }
        }
        n55 = call <vilib>:"Add State(s) to Queue__jki_lib_state_machine.vi"("State(s) in Front (\"\")"="/* Post Error States\n", "State(s) in (\"\")"=w125) -> ("States Out"=w124:string)  [unwired: 13 in]
        "error" <- w121
      }
      frame "Exit" {
        # "Do not put any code in this frame.\n(No errors that occur here will be handled.)"
        n56 = call <vilib>:"Add State(s) to Queue__jki_lib_state_machine.vi"("State(s) in (\"\")"=w135) -> ("States Out"=w134:string)  [unwired: 14 in]
      }
      frame "---------- Data ----------" {
        # "Do not put any code in this frame.\n(It is a separator no-op. You can make a copy of this frame to create a new Data frame)"
        n57 = call <vilib>:"Add State(s) to Queue__jki_lib_state_machine.vi"("State(s) in (\"\")"=w139) -> ("States Out"=w138:string)  [unwired: 14 in]
      }
      frame "Data: Initialize" {
        w140 = TRUE  # fitting enabled
        w141 = TRUE  # fit cursors enabled
        w142 = dbl[] []  # Fit peaks
        w143 = TRUE  # initilize fit
        w144 = dbl[] []  # time offsets
        w145 = TRUE  # Display Error Popup
        w146 = waveform(dbl)[] []  # scopeTraceGUI::1
        w147 = T9 {"Current VI Reference"=refnum, "Close Panel on Exit?"=FALSE}  # Core
        # "Initialize the shift-register data, here.\n(data names are defined by what you wire into the bundle function)"
        n58 = Bundle("Core"=w147, "scopeTraceGUI::1"=w146, "Display Error Popup"=w145, "time offsets"=w144, "initilize fit"=w143, "Fit peaks"=w142, "fit cursors enabled"=w141, "fitting enabled"=w140) -> (w149:T8)  [unwired: 1 in]
        n59 = call <vilib>:"Add State(s) to Queue__jki_lib_state_machine.vi"("State(s) in (\"\")"=w151) -> ("States Out"=w150:string)  [unwired: 14 in]
      }
      frame "Data: Cleanup" {
        # "Cleanup any data and references, here.\n(this is called automatically, by the Macro: Exit)"
        n60 = Unbundle By Name(w152) -> ("Core.Current VI Reference"=w155:refnum<vi>)
        n61 = Close Reference(reference=w155, error in (no error)=w154) -> (error out=w153:errorcluster)
        n62 = call <vilib>:"Add State(s) to Queue__jki_lib_state_machine.vi"("State(s) in (\"\")"=w157) -> ("States Out"=w156:string)  [unwired: 14 in]
      }
      frame "---------- UI ----------" {
        # "Do not put any code in this frame.\n(It is a separator no-op. You can make a copy of this frame to create a new UI frame)"
        n63 = call <vilib>:"Add State(s) to Queue__jki_lib_state_machine.vi"("State(s) in (\"\")"=w161) -> ("States Out"=w160:string)  [unwired: 14 in]
      }
      frame "UI: Initialize" {
        # "Initialize the User Interface, here.\n(this is called automatically, by the Macro: Init)"
        n64 = call <userlib>:"Fit VI window to Largest Dec__ogtk.vi"("error in (no error)"=w163) -> ("error out"=w162:errorcluster)  [unwired: 5 in, 1 out]
        n65 = call <vilib>:"Add State(s) to Queue__jki_lib_state_machine.vi"("State(s) in (\"\")"=w166) -> ("States Out"=w165:string)  [unwired: 14 in]
      }
      frame "UI: ReadFitPar txt" {
        w189 = "Fit width" ("key")
        w204 = "Fit threshold" ("key")
        n66 = call "get software root directory.vi"() -> ("Application Directory"=w219:path)  [unwired: 11 in]
        n67 = Strip Path(path=w219) -> (stripped path=w218:path)  [unwired: 1 out]
        n68 = Build Path(base path=w218, name or relative path="Fit parameters file path") -> (appended path=w217:path)
        n69 = call <vilib>:"Open Config Data.vi"("error in (no error)"=w215, "create file if necessary (T)"=FALSE, "configuration file path"=w217) -> ("error out"=w213:errorcluster, "refnum"=w214:T10)  [unwired: 6 in, 1 out]
        n70 = call-poly <vilib>:"Read Key.vi"("section"=w204, "error in (no error)"=w213, "default value"="", "key"="CH1", "refnum"=w214) -> ("error out"=w226:errorcluster, "value"=w178:string, "found?"=w207:bool, "refnum out"=w227:T10)  [unwired: 3 in]
        n71 = call-poly <vilib>:"Read Key.vi"("section"=w204, "error in (no error)"=w226, "default value"="", "key"="CH2", "refnum"=w227) -> ("error out"=w222:errorcluster, "value"=w179:string, "found?"=w206:bool, "refnum out"=w223:T10)  [unwired: 3 in]
        n72 = call-poly <vilib>:"Read Key.vi"("section"=w204, "error in (no error)"=w222, "default value"="", "key"="CH3", "refnum"=w223) -> ("error out"=w210:errorcluster, "value"=w180:string, "found?"=w205:bool, "refnum out"=w209:T10)  [unwired: 3 in]
        n73 = call-poly <vilib>:"Read Key.vi"("section"=w204, "error in (no error)"=w210, "default value"="", "key"="CH4", "refnum"=w209) -> ("error out"=w188:errorcluster, "value"=w181:string, "found?"=w186:bool, "refnum out"=w187:T10)  [unwired: 3 in]
        n74 = Build Array(w178, w179, w180, w181) -> (w177:string[])
        n75 = Fract/Exp String To Number(string=w177) -> (number=w176:dbl[])  [unwired: 3 in, 1 out]
        n76 = call-poly <vilib>:"Read Key.vi"("section"=w189, "error in (no error)"=w188, "default value"="", "key"="CH1", "refnum"=w187) -> ("error out"=w198:errorcluster, "value"=w174:string, "found?"=w185:bool, "refnum out"=w199:T10)  [unwired: 3 in]
        n77 = call-poly <vilib>:"Read Key.vi"("section"=w189, "error in (no error)"=w198, "default value"="", "key"="CH2", "refnum"=w199) -> ("error out"=w194:errorcluster, "value"=w171:string, "found?"=w184:bool, "refnum out"=w195:T10)  [unwired: 3 in]
        n78 = call-poly <vilib>:"Read Key.vi"("section"=w189, "error in (no error)"=w194, "default value"="", "key"="CH3", "refnum"=w195) -> ("error out"=w191:errorcluster, "value"=w172:string, "found?"=w183:bool, "refnum out"=w190:T10)  [unwired: 3 in]
        n79 = call-poly <vilib>:"Read Key.vi"("section"=w189, "error in (no error)"=w191, "default value"="", "key"="CH4", "refnum"=w190) -> ("error out"=w168:errorcluster, "value"=w173:string, "found?"=w182:bool)  [unwired: 3 in, 1 out]
        n80 = property on="Fit threshold" class="Arr (strict)"(error in=w168, "Val(Sgnl)"=w176) -> (error out=w169:errorcluster)  [unwired: 1 in, 1 out]
        n81 = Compound Arithmetic op=AND(w182, w183, w184, w185, w186, w205, w206, w207) -> (w208:bool)
        n82 = case shown="True" w208 {
          tunnel: [errorcluster {"status"=TRUE, "code"=0, "source"="Stage camera link not found in .txt file"} ("error out") errorcluster {"status"=FALSE, "code"=0, "source"=""} ("error out")] -> w221
          frame False {
          }
          frame True {
          }
        }
        n83 = call <vilib>:"Add State(s) to Queue__jki_lib_state_machine.vi"("State(s) in (\"\")"=w235) -> ("States Out"=w234:string)  [unwired: 14 in]
        n84 = Build Array(w174, w171, w172, w173) -> (w175:string[])
        n85 = Fract/Exp String To Number(string=w175) -> (number=w170:dbl[])  [unwired: 3 in, 1 out]
        n86 = property on="Fit width" class="Arr (strict)"(error in=w169, "Val(Sgnl)"=w170) -> (error out=w167:errorcluster)  [unwired: 1 in, 1 out]
        n87 = Merge Errors(w167, w221) -> (w216:errorcluster)
      }
      frame "UI: Cursor Set" {
        # "Argument"
        # "Set and Unset Cursor Busy.\n(Usage: \"UI: Cursor Set >> Busy|Idle\")"
        n88 = case shown="\"Idle\", Default" w238 {
          tunnel: w240 -> [w245 w247]
          tunnel: [w244 w246] -> w239
          frame "Idle", Default {
            n89 = call <vilib>:"Unset Busy.vi"("error in (no error)"=w245) -> ("error out"=w244:errorcluster)  [unwired: 10 in]
          }
          frame "Busy" {
            n90 = call <vilib>:"Set Busy.vi"("error in (no error)"=w247) -> ("error out"=w246:errorcluster)  [unwired: 9 in, 1 out]
          }
        }
        n91 = call <vilib>:"Add State(s) to Queue__jki_lib_state_machine.vi"("State(s) in (\"\")"=w243) -> ("States Out"=w242:string)  [unwired: 14 in]
      }
      frame "UI: Front Panel State" {
        # "Argument"
        # "Set Front Panel Open or Closed\n(Usage: \"UI: Front Panel State >> Open|Close\")"
        n92 = Unbundle By Name(w250) -> ("Core.Current VI Reference"=w249:refnum<vi>)
        n93 = case shown="\"Open\", Default" w248 {
          tunnel: w252 -> [w258 w271]
          tunnel: [w260 w272] -> w251
          tunnel: w249 -> [w259 w269]
          frame "Open", Default {
            n94 = property class="VI"(reference=w259, error in=w258) -> (reference out=w256:refnum<vi>, error out=w257:errorcluster, "Front Panel.Open"=w255:bool)
            n95 = case shown="False" w255 {
              tunnel: [w263 w266] -> w260
              tunnel: w257 -> [w262 w266]
              tunnel: w256 -> [w261 _]
              frame False {
                n96 = invoke class="VI" method="FP.Open"(reference=w261, error in=w262, "Activate"=TRUE, "State"=T6."Standard") -> (error out=w263:errorcluster)  [unwired: 1 in, 4 out]
              }
              frame True {
              }
            }
          }
          frame "Close" {
            n97 = property class="VI"(reference=w269, error in=w271) -> (reference out=w268:refnum<vi>, error out=w270:errorcluster, "Front Panel.Open"=w267:bool)
            n98 = case shown="True" w267 {
              tunnel: [w273 w276] -> w272
              tunnel: w270 -> [w273 w275]
              tunnel: w268 -> [_ w274]
              frame False {
              }
              frame True {
                n99 = invoke class="VI" method="FP.Close"(reference=w274, error in=w275) -> (error out=w276:errorcluster)  [unwired: 1 in, 2 out]
              }
            }
          }
        }
        n100 = call <vilib>:"Add State(s) to Queue__jki_lib_state_machine.vi"("State(s) in (\"\")"=w254) -> ("States Out"=w253:string)  [unwired: 14 in]
      }
      frame "---------- Macro ----------" {
        # "Do not put any code in this frame.\n(It is a separator no-op. You can make a copy of this frame to create a new Macro frame)"
        n101 = call <vilib>:"Add State(s) to Queue__jki_lib_state_machine.vi"("State(s) in (\"\")"=w280) -> ("States Out"=w279:string)  [unwired: 14 in]
      }
      frame "Macro: Initialize" {
        w281 = "Data: Initialize\nInitialize Core Data\nUI: Initialize\nUI: ReadFitPar txt\nUI: Front Panel State >> Open"  # Data: Initialize Initialize Core Data UI: Initialize UI: ReadFitPar txt UI: Front Panel State >> Open
        # "Initialization Macro\n(This is called once, when the VI starts)"
        n102 = call <vilib>:"Add State(s) to Queue__jki_lib_state_machine.vi"("State(s) in Front (\"\")"=w281, "State(s) in (\"\")"=w285) -> ("States Out"=w284:string)  [unwired: 13 in]
      }
      frame "Macro: Exit" {
        # "Exit Macro\n(This is called once, when the VI exits)"
        n103 = Unbundle By Name(w293) -> ("Core.Close Panel on Exit?"=w292:bool)
        n104 = Select(t="UI: Front Panel State >> Close", s=w292, f="") -> (s? t:f=w289:string)
        n105 = call <vilib>:"Add State(s) to Queue__jki_lib_state_machine.vi"("State(s) in (\"\")"=w289, "State(s) at Back (\"\")"="Data: Cleanup\nExit") -> ("States Out"=w287:string)  [unwired: 13 in]
        n106 = call <vilib>:"Add State(s) to Queue__jki_lib_state_machine.vi"("State(s) in Front (\"\")"=w287, "State(s) in (\"\")"=w295) -> ("States Out"=w294:string)  [unwired: 13 in]
      }
      frame "---------- Actions ----------" {
        n107 = call <vilib>:"Add State(s) to Queue__jki_lib_state_machine.vi"("State(s) in (\"\")"=w299) -> ("States Out"=w298:string)  [unwired: 14 in]
      }
      frame "Action: correct timescale & update plot" {
        # "Change both the label of the \n\"Channel\" & \"ScopeTraceGUI\"\nto connect to the right device"
        n108 = Unbundle By Name("Digitizer Traces") -> ("scopeTraceGUI::1"=w303:waveform(dbl)[])
        n109 = Unbundle By Name(w302) -> ("scopeTraceGUI::1"=w309:waveform(dbl)[])
        n110 = Not Equal?(x=w309, y=w303) -> (x != y?=w308:bool)
        n111 = Index Array(array=w303) -> (element=w307:waveform(dbl))  [unwired: 1 in]
        n112 = call-poly <vilib>:"Waveform Duration.vi"("waveform in"=w307) -> ("duration"=w306:dbl)  [unwired: 8 in, 2 out]
        "duration" <- w306
        n113 = Greater Than 0?(x=w306) -> (x > 0?=w305:bool)
        n114 = Compound Arithmetic op=AND(w308, w305) -> (w304:bool)
        n115 = case shown="True" w304 {
          tunnel: [w316 w318] -> w312
          tunnel: w303 -> [_ w328]
          tunnel: w302 -> [w316 w320]
          tunnel: w311 -> [w315 w327]
          tunnel: [w315 w326] -> w310
          tunnel: [_ ""] -> w300
          frame False {
          }
          frame True {
            n116 = Build Array("value3::2", "value4::2", "value5::2", "value6::2") -> (w321:dbl[])
            n117 = for {
              tunnel: w328 -> [w332] mode=indexing
              tunnel: w321 -> [w330] mode=indexing
              tunnel: [w334] -> w319 mode=indexing
              tunnel: w327 -> [w333]
              tunnel: [w333] -> w326
              n118 = Unbundle By Name(w332) -> ("t0"=w331:timestamp)
              n119 = Add(x=w331, y=w330) -> (x+y=w329:timestamp)
              n120 = Bundle By Name(cluster=w332, "t0"=w329) -> (w334:waveform(dbl))
            }
            "all traces" <- w319
            n121 = Bundle By Name(cluster=w320, "time offsets"=w321, "scopeTraceGUI::1"=w319) -> (w318:T8)
          }
        }
        n122 = call <vilib>:"Add State(s) to Queue__jki_lib_state_machine.vi"("State(s) in Front (\"\")"=w300, "State(s) in (\"\")"=w314) -> ("States Out"=w313:string)  [unwired: 13 in]
      }
      frame "Action: Fit" {
        n123 = Unbundle By Name(w341) -> ("time offsets"=w345:dbl[], "scopeTraceGUI::1"=w344:waveform(dbl)[], "initilize fit"=w342:bool)
        n124 = for {
          tunnel: w345 -> [w359] mode=indexing
          tunnel: w344 -> [w358] mode=indexing
          tunnel: [w357] -> w336 mode=indexing
          tunnel: [w356] -> w343 mode=indexing
          tunnel: w342 -> [w355]
          tunnel: "Fit threshold" -> [w354] mode=indexing
          tunnel: "Fit width" -> [w353] mode=indexing
          tunnel: "Type" -> [w348] mode=indexing
          n125 = Unbundle By Name(w358) -> ("dt"=w351:dbl, "Y"=w349:dbl[])
          n126 = case shown="\"Threshold\"" w348 {
            tunnel: [w369 _] -> w356
            tunnel: w355 -> [w368 _]
            tunnel: w354 -> [w367 w370]
            tunnel: w353 -> [w366 _]
            tunnel: [w365 w372] -> w350
            tunnel: w349 -> [w362 w371]
            frame "Peak fit", Default {
              n127 = call <vilib>:"Peak Detector.vi"("initialize (T)"=w368, "peaks/valleys"=enum32{"Peaks", "Valleys"}."Peaks", "width"=w366, "threshold"=w367, "X"=w362) -> ("Amplitudes"=w361:dbl[], "Locations"=w363:dbl[], "# found"=w369:i32)  [unwired: 2 in, 2 out]
              n128 = Array Max & Min(array=w361) -> (max index (indices)=w364:i32)  [unwired: 3 out]
              n129 = Index Array(array=w363, index=w364) -> (element=w365:dbl)
            }
            frame "Threshold" {
              n130 = Threshold 1D Array(2:w370, 3:w371) -> (0:w372:dbl)  [unwired: 1 in]
            }
          }
          n131 = Multiply(x=w351, y=w350) -> (x*y=w352:dbl)
          n132 = Add(x=w359, y=w352) -> (x+y=w357:dbl)
        }
        "Time of peak" <- w336
        "Number of peaks found" <- w343
        n133 = disable-structure shown="Disabled" {
          frame Disabled {
            n134 = call-poly <vilib>:"Amplitude and Levels.vi"() -> ()  [unwired: 8 in, 4 out]
            n135 = call-poly <vilib>:"Pulse Measurements.vi"() -> ()  [unwired: 7 in, 5 out]
          }
          frame Enabled {
          }
        }
        n136 = Bundle By Name(cluster=w341, "initilize fit"=FALSE, "Fit peaks"=w336) -> (w340:T8)
      }
      frame "Action: update fit cursors" {
        n137 = Unbundle By Name(w375) -> ("Fit peaks"=w376:dbl[])
        n138 = for {
          shift-right: [w380] -> w373
          shift-left: w374 -> [w381]
          tunnel: w376 -> [w378] mode=indexing
          i -> [w379]
          n139 = property on="all traces" class="WFGraph (strict)"(error in=w381, "Active Cursor"=w379, "Cursor.Cursor X"=w378) -> (error out=w380:errorcluster)  [unwired: 1 in, 1 out]
        }
      }
      frame "Action: enable fit cursors" {
        n140 = Unbundle By Name(w387) -> ("fit cursors enabled"=w385:bool, "fitting enabled"=w382:bool)
        n141 = property on="800nm w.r.t. 532nm" class="DigNum (strict)"(error in=w384, "Visible"=w382) -> (error out=w386:errorcluster)  [unwired: 1 in, 1 out]
        n142 = property on="800nm w.r.t. Discharge (mean)" class="DigNum (strict)"(error in=w386, "Visible"=w382) -> (error out=w383:errorcluster)  [unwired: 1 in, 1 out]
        n143 = case shown="False" w385 {
          tunnel: w383 -> [w391 w394]
          tunnel: [w390 w393] -> w389
          frame False {
            n144 = property on="all traces" class="WFGraph (strict)"(error in=w391, "CrsrList"=T7 [] ("Cursor List 2")) -> (error out=w390:errorcluster)  [unwired: 1 in, 1 out]
          }
          frame True {
            n145 = property on="all traces" class="WFGraph (strict)"(error in=w394, "CrsrList"=T7 [{"Name"="Fit CH1", "Color"=16448250, "Style"=2, "Point Style"=10, "Name Visible"=FALSE, "Allow Drag"=TRUE, "Cursor Mode"=0, "Plot"=0, "Index"=2, "Position"={"X"=0.0, "Y"=-1000.0}, "X Scale"=0, "Y Scale"=0, "Watch Plots"=[], "Watch All Plots"=FALSE, "Plot Area"=0, "Label Offset"={"X"=0.0, "Y"=0.0}}, {"Name"="Fit CH2", "Color"=16711680, "Style"=2, "Point Style"=10, "Name Visible"=FALSE, "Allow Drag"=TRUE, "Cursor Mode"=0, "Plot"=0, "Index"=0, "Position"={"X"=0.0, "Y"=-1000.0}, "X Scale"=0, "Y Scale"=0, "Watch Plots"=[], "Watch All Plots"=FALSE, "Plot Area"=0, "Label Offset"={"X"=0.0, "Y"=0.0}}, {"Name"="Fit CH3", "Color"=6618880, "Style"=2, "Point Style"=10, "Name Visible"=FALSE, "Allow Drag"=TRUE, "Cursor Mode"=0, "Plot"=0, "Index"=0, "Position"={"X"=0.0, "Y"=-1000.0}, "X Scale"=0, "Y Scale"=0, "Watch Plots"=[], "Watch All Plots"=FALSE, "Plot Area"=0, "Label Offset"={"X"=0.0, "Y"=0.002228412256267409}}, {"Name"="Fit CH4", "Color"=3381759, "Style"=2, "Point Style"=10, "Name Visible"=FALSE, "Allow Drag"=TRUE, "Cursor Mode"=0, "Plot"=0, "Index"=0, "Position"={"X"=0.0, "Y"=-1000.0}, "X Scale"=0, "Y Scale"=0, "Watch Plots"=[], "Watch All Plots"=FALSE, "Plot Area"=0, "Label Offset"={"X"=0.0, "Y"=0.002228412256267409}}] ("Cursor List 2")) -> (error out=w393:errorcluster)  [unwired: 1 in, 1 out]
          }
        }
      }
      frame "Action: Calculate timings" {
        n146 = Unbundle By Name(w406) -> ("Fit peaks"=w405:dbl[])
        n147 = Index Array(array=w405) -> (element #1=w404:dbl, element #2=w398:dbl, element #3=w401:dbl, element #4=w402:dbl)  [unwired: 4 in]
        n148 = Add(x=w401, y=w402) -> (x+y=w400:dbl)
        n149 = Subtract(x=w398, y=w404) -> (x-y=→"800nm w.r.t. 532nm":dbl)
        n150 = Divide(x=w400, y=2.0) -> (x/y=w397:dbl)
        n151 = Subtract(x=w398, y=w397) -> (x-y=→"800nm w.r.t. Discharge (mean)":dbl)
      }
      frame "Action: adjust scaling" {
        n152 = Not(x="graph") -> (.not. x?=w410:bool)
        n153 = property on="Channel to scale" class="Ring (strict)"(error in=w411, "Visible"=w410) -> (error out=w412:errorcluster)  [unwired: 1 in, 1 out]
        n154 = for {
          N: 4 -> [_]
          tunnel: [w456] -> w421 mode=indexing
          tunnel: [w455] -> w420 mode=indexing
          i -> [w457]
          n155 = case shown="0, Default" w457 {
            tunnel: ["Verticalrange.Channel0::1" "Verticalrange.Channel1::1" "Verticalrange.Channel2::1" "Verticalrange.Channel3::1"] -> w463
            tunnel: [w469 w473 w480 w487] -> w460
            frame 0, Default {
              n156 = Select(t=-1.0 ("y"), s="CH 1:", f=1.0 ("y")) -> (s? t:f=w466:dbl)
              n157 = Multiply(x="Verticaloffset.Channel0::1", y=w466) -> (x*y=w469:dbl)
            }
            frame 1 {
              n158 = Select(t=-1.0 ("y"), s="CH 2:", f=1.0 ("y")) -> (s? t:f=w474:dbl)
              n159 = Multiply(x="Verticaloffset.Channel1::1", y=w474) -> (x*y=w473:dbl)
            }
            frame 2 {
              n160 = Select(t=-1.0 ("y"), s="CH 3:", f=1.0 ("y")) -> (s? t:f=w483:dbl)
              n161 = Multiply(x="Verticaloffset.Channel2::1", y=w483) -> (x*y=w480:dbl)
            }
            frame 3 {
              n162 = Select(t=-1.0 ("y"), s="CH 4:", f=1.0 ("y")) -> (s? t:f=w488:dbl)
              n163 = Multiply(x="Verticaloffset.Channel3::1", y=w488) -> (x*y=w487:dbl)
            }
          }
          n164 = Divide(x=w463, y=2.0) -> (x/y=w459:dbl)
          n165 = Multiply(x=w459, y=-1.0) -> (x*y=w458:dbl)
          n166 = Subtract(x=w458, y=w460) -> (x-y=w456:dbl)
          n167 = Subtract(x=w459, y=w460) -> (x-y=w455:dbl)
        }
        n168 = Select(t="main_graph", s="graph", f="raw_graph") -> (s? t:f=w413:string)
        n169 = case shown="\"raw_graph\", Default" w413 {
          tunnel: w421 -> [w449 w454]
          tunnel: w420 -> [w448 w453]
          tunnel: [w439 w452] -> w419
          tunnel: [w438 w451] -> w418
          tunnel: [w435 _] -> w417
          tunnel: [w437 _] -> w416
          frame "main_graph" {
            n170 = Index Array(array=w448) -> (element #1=w443:dbl, element #2=w442:dbl, element #3=w441:dbl, element #4=w440:dbl)  [unwired: 4 in]
            n171 = Index Array(array=w449) -> (element #1=w447:dbl, element #2=w446:dbl, element #3=w445:dbl, element #4=w444:dbl)  [unwired: 4 in]
            n172 = Max & Min(x=w447, y=w446) -> (min(x,y)=w439:dbl)  [unwired: 1 out]
            n173 = Max & Min(x=w445, y=w444) -> (min(x,y)=w434:dbl)  [unwired: 1 out]
            n174 = Max & Min(x=w443, y=w442) -> (max(x,y)=w438:dbl)  [unwired: 1 out]
            n175 = Max & Min(x=w441, y=w440) -> (max(x,y)=w436:dbl)  [unwired: 1 out]
            n176 = Multiply(x=w434, y=10.0) -> (x*y=w435:dbl)
            n177 = Multiply(x=w436, y=10.0) -> (x*y=w437:dbl)
          }
          frame "raw_graph", Default {
            n178 = Index Array(array=w454, index="Channel to scale") -> (element=w452:dbl)
            n179 = Index Array(array=w453, index="Channel to scale") -> (element=w451:dbl)
          }
        }
        n180 = Multiply(x="TimeAxis.Time base::1", y=10.0) -> (x*y=w423:dbl)
        n181 = case shown="\"main_graph\"" w413 {
          tunnel: u8 0 ("Y Scale.Scale Fit") -> [w497 w512]
          tunnel: u8 0 ("X Scale.Scale Fit") -> [w500 w511]
          tunnel: 0.0 ("X Scale.Range:Minimum") -> [w502 w510]
          tunnel: [w503 w509] -> w428
          tunnel: w412 -> [w504 w508]
          tunnel: w423 -> [w501 w507]
          tunnel: w419 -> [w499 w506]
          tunnel: w418 -> [w498 w505]
          tunnel: w417 -> [w493 _]
          tunnel: w416 -> [w492 _]
          frame "main_graph" {
            n182 = property on="all traces" class="WFGraph (strict)"(error in=w504, "XScale.Minimum"=w502, "XScale.Maximum"=w501, "XScale.ScaleFit"=w500, "ActYScl"=1 ("Active Y Scale"), "YScale.Minimum"=w499, "YScale.Maximum"=w498, "YScale.ScaleFit"=w497, "ActYScl"=0 ("Active Y Scale"), "YScale.Minimum"=w493, "YScale.Maximum"=w492, "YScale.ScaleFit"=u8 0 ("Y Scale.Scale Fit")) -> (error out=w503:errorcluster)  [unwired: 1 in, 1 out]
          }
          frame "raw_graph", Default {
            n183 = property on="scopeTraceGUI::1" class="WFGraph (strict)"(error in=w508, "XScale.Minimum"=w510, "XScale.Maximum"=w507, "XScale.ScaleFit"=w511, "YScale.Minimum"=w506, "YScale.Maximum"=w505, "YScale.ScaleFit"=w512) -> (error out=w509:errorcluster)  [unwired: 1 in, 1 out]
          }
        }
      }
    }
  }
  n184 = call "GUI_Master_subvi_reentrant_queues.vi"("STOP Queue in"=w6, "This Application"=w11, "error in (no error)"=w12, "tcp data event"=w10, "Caller menu reference"=w14, "Caller VI ref"=w15) -> ("error out"=→"error IO 2":errorcluster)  [unwired: 5 in]
  n185 = Unregister For Events(event registration refnum=w7, error in=w4) -> (error out=w5:errorcluster)
  n186 = Release Queue(queue=w6, error in (no error)=w4) -> ()  [unwired: 1 in, 3 out]
  n187 = Destroy User Event(user event=w10, error in=w5) -> ()  [unwired: 1 out]
